vi "Read GIF File (Animated) Example.vi"() -> ()   [LabVIEW 2011]
panel:
  out "Array":u32[][][](array[colorbox])
  in  "path to GIF file":path
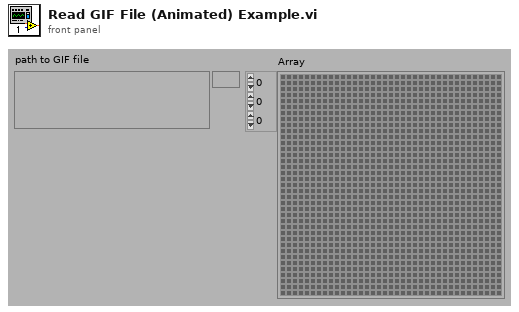
[diagram p1: front panel]
types:
  T1 = typedef "imagedata.ctl" = cluster{"image type":i32, "image depth":i32, "image":u8[], "mask":u8[], "colors":u32[], "Rectangle":cluster{"left":i16, "top":i16, "right":i16, "bottom":i16}}
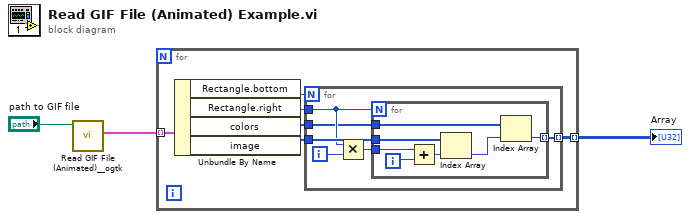
[diagram p0: block diagram]
diagram:
  n1 = call <userlib>:"Read GIF File (Animated)__ogtk.vi"("path to GIF file"="path to GIF file") -> ("images data"=w2:T1[])  [unwired: 6 in, 4 out]
  n2 = for {
    tunnel: w2 -> [w9] mode=indexing
    tunnel: [w8] -> w1 mode=indexing
    n3 = Unbundle By Name(w9) -> ("Rectangle.bottom"=w7:i16, "Rectangle.right"=w6:i16, "colors"=w4:u32[], "image"=w5:u8[])
    n4 = for {
      N: w7 -> [_]
      tunnel: w6 -> [w13]
      tunnel: w5 -> [w15]
      tunnel: w4 -> [w11]
      tunnel: [w10] -> w8 mode=indexing
      i -> [w14]
      n5 = Multiply(x=w13, y=w14) -> (x*y=w12:i32)
      n6 = for {
        N: w13 -> [_]
        tunnel: w15 -> [w22]
        tunnel: w12 -> [w21]
        tunnel: w11 -> [w18]
        tunnel: [w16] -> w10 mode=indexing
        i -> [w20]
        n7 = Add(x=w21, y=w20) -> (x+y=w19:i32)
        n8 = Index Array(array=w22, index=w19) -> (element=w17:u8)
        n9 = Index Array(array=w18, index=w17) -> (element=w16:u32)
      }
    }
  }
  "Array" <- w1
